vi "test_full_flow.vi"() -> ()   [LabVIEW 2020, in "reqwest_tests.lvlib"]
uses:
  reqwest_tests.lvlib
  <vilib>/addons/_JKI Toolkits/Caraya/classes/Assert/Assert.lvclass
  <vilib>/addons/_JKI Toolkits/Caraya/classes/Test/Test.lvclass
  ClientBuilder/ClientBuilder.lvclass
  Client/Client.lvclass
  Headers/Headers.lvclass
  Request/Request.lvclass
panel:
  out "is_complete":bool
  out "string_value":string
  in  "error in (no error)":errorcluster
  out "error out":errorcluster
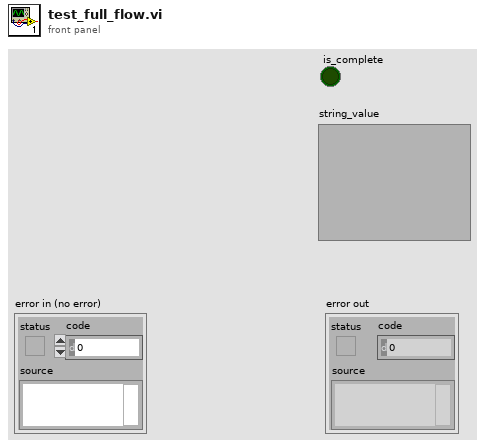
[diagram p1: front panel]
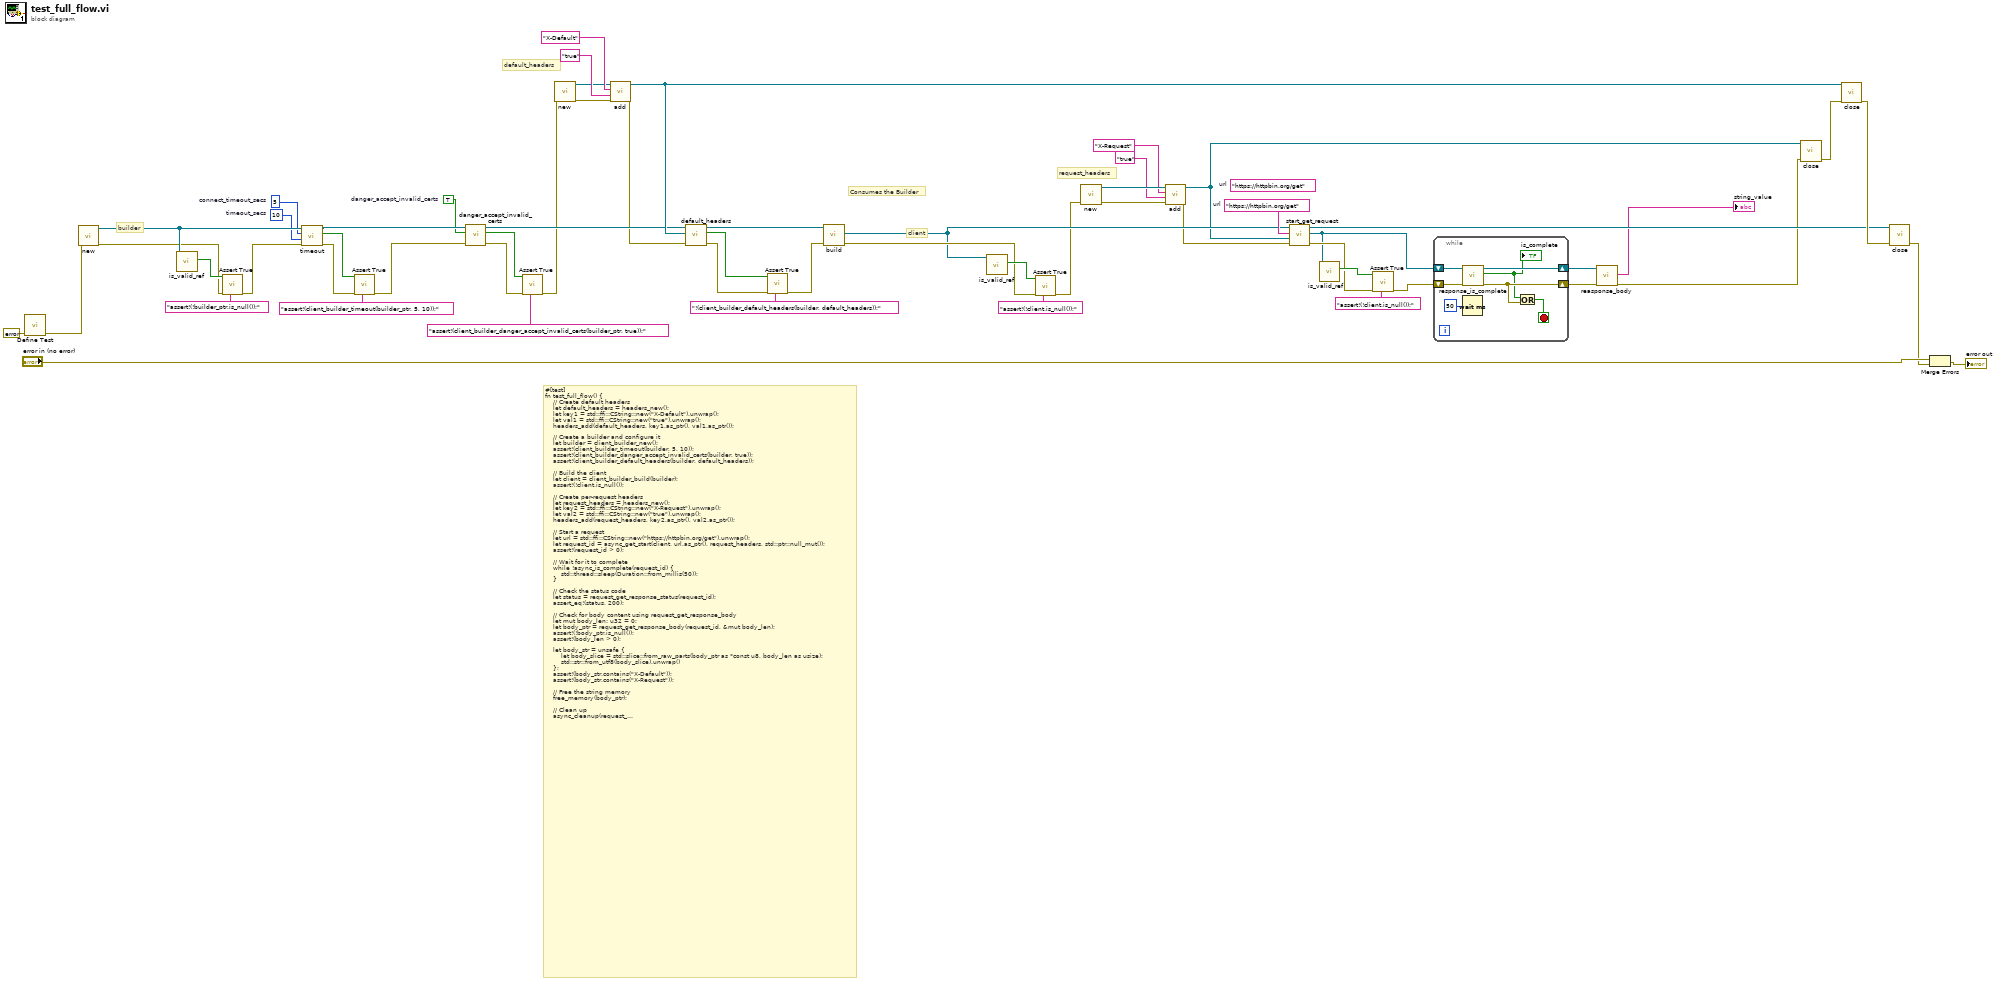
[diagram p0: block diagram]
diagram:
  (unwired) "https://httpbin.org/get"  # url
  w19 = "https://httpbin.org/get"  # url
  w47 = TRUE  # danger_accept_invalid_certs
  w51 = u64 10  # timeout_secs
  w52 = u64 5  # connect_timeout_secs
  # "request_headers"
  # "client"
  # "default_headers"
  # "builder"
  # "Consumes the Builder"
  # "#[test]\nfn test_full_flow() {\n    // Create default headers\n    let default_headers = headers_new();\n    let key1 = std::ffi::CString::new(\"X-Default\").unwrap();\n    let val1 = std::ffi::CString::new(\"true\").unwrap();\n    headers_add(default_headers, key1.as_ptr(), val1.as_ptr());\n\n    // Create a builder and configure it\n    let builder = client_builder_new();\n    assert!(client_builder_timeout(builder, 5, 10));\n    assert!(client_builder_danger_accept_invalid_certs(builder, true));\n    assert!(client_builder_default_headers(builder, default_headers));\n\n    // Build the client\n    let client = client_builder_build(builder);\n    assert!(!client.is_null());\n\n    // Create per-request headers\n    let request_headers = headers_new();\n    let key2 = std::ffi::CString::new(\"X-Request\").unwrap();\n    let val2 = std::ffi::CString::new(\"true\").unwrap();\n    headers_add(request_headers, key2.as_ptr(), val2.as_ptr());\n\n    // Start a request\n    let url = std::ffi::CString::new(\"https://httpbin.org/get\").unwrap();\n    let request_id = async_get_start(client, url.as_ptr(), request_headers, std::ptr::null_mut());\n    assert!(request_id > 0);\n\n    // Wait for it to complete\n    while !async_is_complete(request_id) {\n        std::thread::sleep(Duration::from_millis(50));\n    }\n\n    // Check the status code\n    let status = request_get_response_status(request_id);\n    assert_eq!(status, 200);\n\n    // Check for body content using request_get_response_body\n    let mut body_len: u32 = 0;\n    let body_ptr = request_get_response_body(request_id, &mut body_len);\n    assert!(!body_ptr.is_null());\n    assert!(body_len > 0);\n\n    let body_str = unsafe {\n        let body_slice = std::slice::from_raw_parts(body_ptr as *const u8, body_len as usize);\n        std::str::from_utf8(body_slice).unwrap()\n    };\n    assert!(body_str.contains(\"X-Default\"));\n    assert!(body_str.contains(\"X-Request\"));\n\n    // Free the string memory\n    free_memory(body_ptr);\n\n    // Clean up\n    async_cleanup(request_id);\n    headers_free(request_headers);\n    headers_free(default_headers);\n    client_close(client);\n}"
  n1 = call <vilib>:"Define Test.vi"("error in (no error)"=errorcluster {"status"=FALSE, "code"=0, "source"=""}) -> ("error out"=w41:errorcluster)  [unwired: 9 in, 1 out]
  n2 = call "new.vi"("error in (no error)"=w41) -> ("error out"=w40:errorcluster, "Client out"=w53:refnum<class "ClientBuilder.lvclass">)  [unwired: 9 in]
  n3 = call "is_valid_ref.vi"("Client in"=w53) -> ("valid-ref?"=w55:bool)  [unwired: 10 in]
  n4 = call <vilib>:"Assert True.vi"("Label"="assert!(!builder_ptr.is_null());", "error in (no error)"=w40, "True?"=w55) -> ("error out"=w39:errorcluster)  [unwired: 7 in, 1 out]
  n5 = call "timeout.vi"("error in (no error)"=w39, "timeout_secs"=w51, "connect_timeout_secs"=w52, "ClientBuilder in"=w53) -> ("error out"=w38:errorcluster, "success"=w49:bool, "ClientBuilder out"=w48:refnum<class "ClientBuilder.lvclass">)  [unwired: 5 in]
  n6 = call <vilib>:"Assert True.vi"("Label"="assert!(client_builder_timeout(builder_ptr, 5, 10));", "error in (no error)"=w38, "True?"=w49) -> ("error out"=w37:errorcluster)  [unwired: 7 in, 1 out]
  n7 = call "danger_accept_invalid_certs.vi"("error in (no error)"=w37, "danger_accept_invalid_certs"=w47, "ClientBuilder in"=w48) -> ("error out"=w36:errorcluster, "success"=w45:bool, "ClientBuilder out"=w29:refnum<class "ClientBuilder.lvclass">)  [unwired: 6 in]
  n8 = call <vilib>:"Assert True.vi"("Label"="assert!(client_builder_danger_accept_invalid_certs(builder_ptr, true));", "error in (no error)"=w36, "True?"=w45) -> ("error out"=w13:errorcluster)  [unwired: 7 in, 1 out]
  n9 = call "new.vi"("error in (no error)"=w13) -> ("error out"=w31:errorcluster, "Headers out"=w32:refnum<class "Headers.lvclass">)  [unwired: 9 in]
  n10 = call "add.vi"("error in (no error)"=w31, "value"="true", "key"="X-Default", "Headers in"=w32) -> ("error out"=w12:errorcluster, "Headers out"=w30:refnum<class "Headers.lvclass">)  [unwired: 5 in, 1 out]
  n11 = call "default_headers.vi"("error in (no error)"=w12, "Headers"=w30, "ClientBuilder in"=w29) -> ("error out"=w26:errorcluster, "success"=w27:bool, "ClientBuilder out"=w28:refnum<class "ClientBuilder.lvclass">)  [unwired: 6 in]
  n12 = call <vilib>:"Assert True.vi"("Label"="!(client_builder_default_headers(builder, default_headers));", "error in (no error)"=w26, "True?"=w27) -> ("error out"=w25:errorcluster)  [unwired: 7 in, 1 out]
  n13 = call "build.vi"("error in (no error)"=w25, "ClientBuilder in"=w28) -> ("error out"=w35:errorcluster, "Client out"=w18:refnum<class "Client.lvclass">)  [unwired: 8 in]
  n14 = call "is_valid_ref.vi"("Client in"=w18) -> ("valid-ref?"=w44:bool)  [unwired: 10 in]
  n15 = call <vilib>:"Assert True.vi"("Label"="assert!(!client.is_null());", "error in (no error)"=w35, "True?"=w44) -> ("error out"=w9:errorcluster)  [unwired: 7 in, 1 out]
  n16 = call "new.vi"("error in (no error)"=w9) -> ("error out"=w23:errorcluster, "Headers out"=w22:refnum<class "Headers.lvclass">)  [unwired: 9 in]
  n17 = call "add.vi"("error in (no error)"=w23, "value"="true", "key"="X-Request", "Headers in"=w22) -> ("error out"=w8:errorcluster, "Headers out"=w14:refnum<class "Headers.lvclass">)  [unwired: 5 in, 1 out]
  n18 = call "start_get_request.vi"("error in (no error)"=w8, "Headers in"=w14, "url"=w19, "Client in"=w18) -> ("error out"=w15:errorcluster, "Request"=w6:refnum<class "Request.lvclass">, "Client out"=w7:refnum<class "Client.lvclass">)  [unwired: 5 in]
  n19 = call "is_valid_ref.vi"("Request in"=w6) -> ("valid-ref?"=w16:bool)  [unwired: 10 in]
  n20 = call <vilib>:"Assert True.vi"("Label"="assert!(!client.is_null());", "error in (no error)"=w15, "True?"=w16) -> ("error out"=w5:errorcluster)  [unwired: 7 in, 1 out]
  n21 = while {
    shift-right: [w65] -> w1
    shift-left: w6 -> [w64]
    shift-right: [w61] -> w4
    shift-left: w5 -> [w62]
    stop <- w59 stop-if-true
    n22 = Wait (ms)(milliseconds to wait=u32 50) -> ()  [unwired: 1 out]
    n23 = call "response_is_complete.vi"("error in (no error)"=w62, "Request in"=w64) -> ("error out"=w61:errorcluster, "is_complete"=w60:bool, "Request out"=w65:refnum<class "Request.lvclass">)  [unwired: 7 in]
    "is_complete" <- w60
    n24 = Or(x=w60, y=w61) -> (x .or. y?=w59:bool)
  }
  n25 = call "reasponse_body.vi"("error in (no error)"=w4, "Request in"=w1) -> ("error out"=w3:errorcluster, "string_value"=→"string_value":string)  [unwired: 7 in, 1 out]
  n26 = call "close.vi"("error in (no error)"=w3, "Headers in"=w14) -> ("error out"=w11:errorcluster)  [unwired: 9 in]
  n27 = call "close.vi"("error in (no error)"=w11, "Headers in"=w30) -> ("error out"=w10:errorcluster)  [unwired: 9 in]
  n28 = call "close.vi"("error in (no error)"=w10, "Client in"=w7) -> ("error out"=w42:errorcluster)  [unwired: 9 in]
  n29 = Merge Errors("error in (no error)", w42) -> (→"error out":errorcluster)
